vi "Create Clean Task.vi"(8 "error in":errorcluster, 11 "4300 in":refnum<class "4300.lvclass">) -> (0 "error out":errorcluster, 3 "4300 out":refnum<class "4300.lvclass">)   [LabVIEW 2019, in "4300.lvlib" / "4300.lvclass"]
uses:
  Library/4300.lvclass
  C:/Users/Public/Documents/Development/builds/Instruments/Instruments.lvlibp/Library/Instruments.lvclass
  Library/4300.lvclass/4300.ctl
  builds/Instruments/Instruments.lvlibp/Accessors/Read Resource.vi
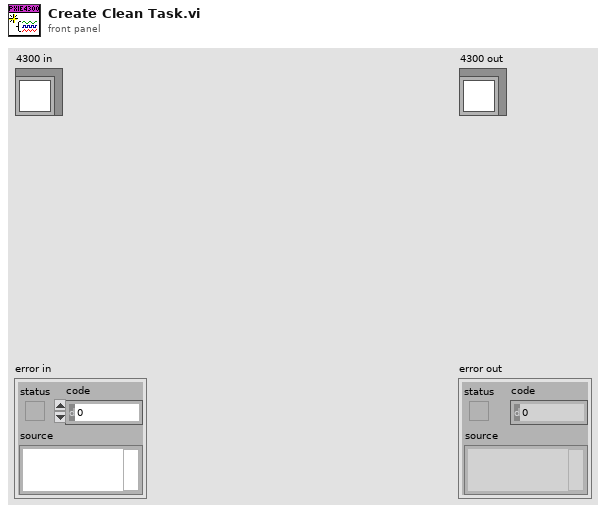
[diagram p1: front panel]
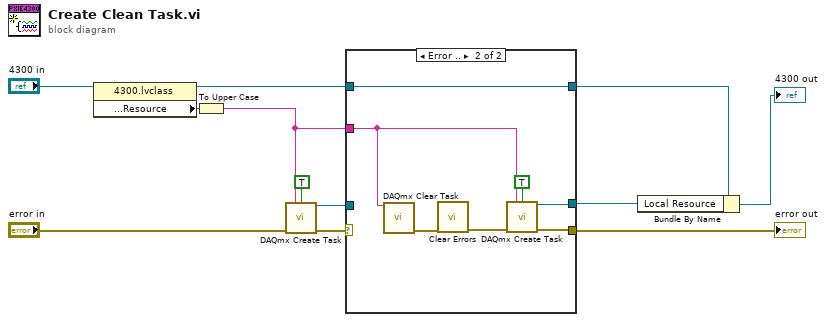
[diagram p0: block diagram]
diagram:
  n1 = property class="4300.lvclass"(reference="4300 in") -> (reference out=w4:refnum<class "4300.lvclass">, "Accessors:Configuration:Resource"=w6:string)  [unwired: 1 in, 1 out]
  n2 = To Upper Case(1:w6) -> (0:w5:string)
  n3 = call <vilib>:"DAQmx Create Task.vi"("new task name"=w5, "auto cleanup"=TRUE, "error in"="error in") -> ("task out"=w12:refnum<k21>, "error out"=w11:errorcluster)  [unwired: 11 in]
  n4 = case shown="Error .." w11 {
    selector: w11 -> [w15 _]
    tunnel: [w15 w20] -> w9
    tunnel: w12 -> [w14 _]
    tunnel: w5 -> [_ w18]
    tunnel: [w14 w19] -> w1
    tunnel: w4 -> [w13 w16]
    tunnel: [w13 w16] -> w3
    frame No Error {
    }
    frame Error {
      n5 = call <vilib>:"DAQmx Clear Task.vi"("task in"=w18) -> ("error out"=w22:errorcluster)  [unwired: 14 in]
      n6 = call <vilib>:"Clear Errors.vi"("error in (no error)"=w22) -> ("error out"=w21:errorcluster)  [unwired: 5 in, 1 out]
      n7 = call <vilib>:"DAQmx Create Task.vi"("new task name"=w18, "auto cleanup"=TRUE, "error in"=w21) -> ("task out"=w19:refnum<k21>, "error out"=w20:errorcluster)  [unwired: 11 in]
    }
  }
  "error out" <- w9
  n8 = Bundle By Name(cluster=w3, "Local Resource"=w1) -> (→"4300 out":refnum<class "4300.lvclass">)
